vi "interface.vi"() -> ()   [LabVIEW 2016, in "Alarm interface.lvlib"]
uses:
  Alarm interface.lvlib
  WxMessage/wxpusher.lvlib
panel:
  in  "短信/语音设置":bool
  in  "微信设置":bool
  in  "报警定义":bool
  out "报警内容":string
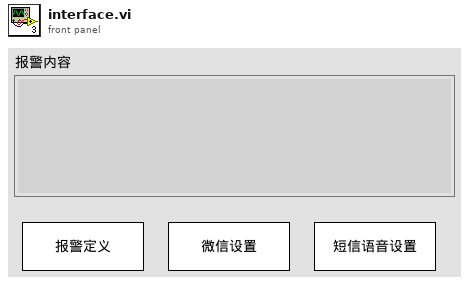
[diagram p1: front panel]
types:
  T1 = cluster{"报警模块":string, "告警码":string, "告警内容":string}
  T2 = enum32{"Invalid", "Standard", "Closed", "Hidden", "Minimized", "Maximized"}
  T3 = enum32{"Bad", "Idle", "Run top level", "Running"}
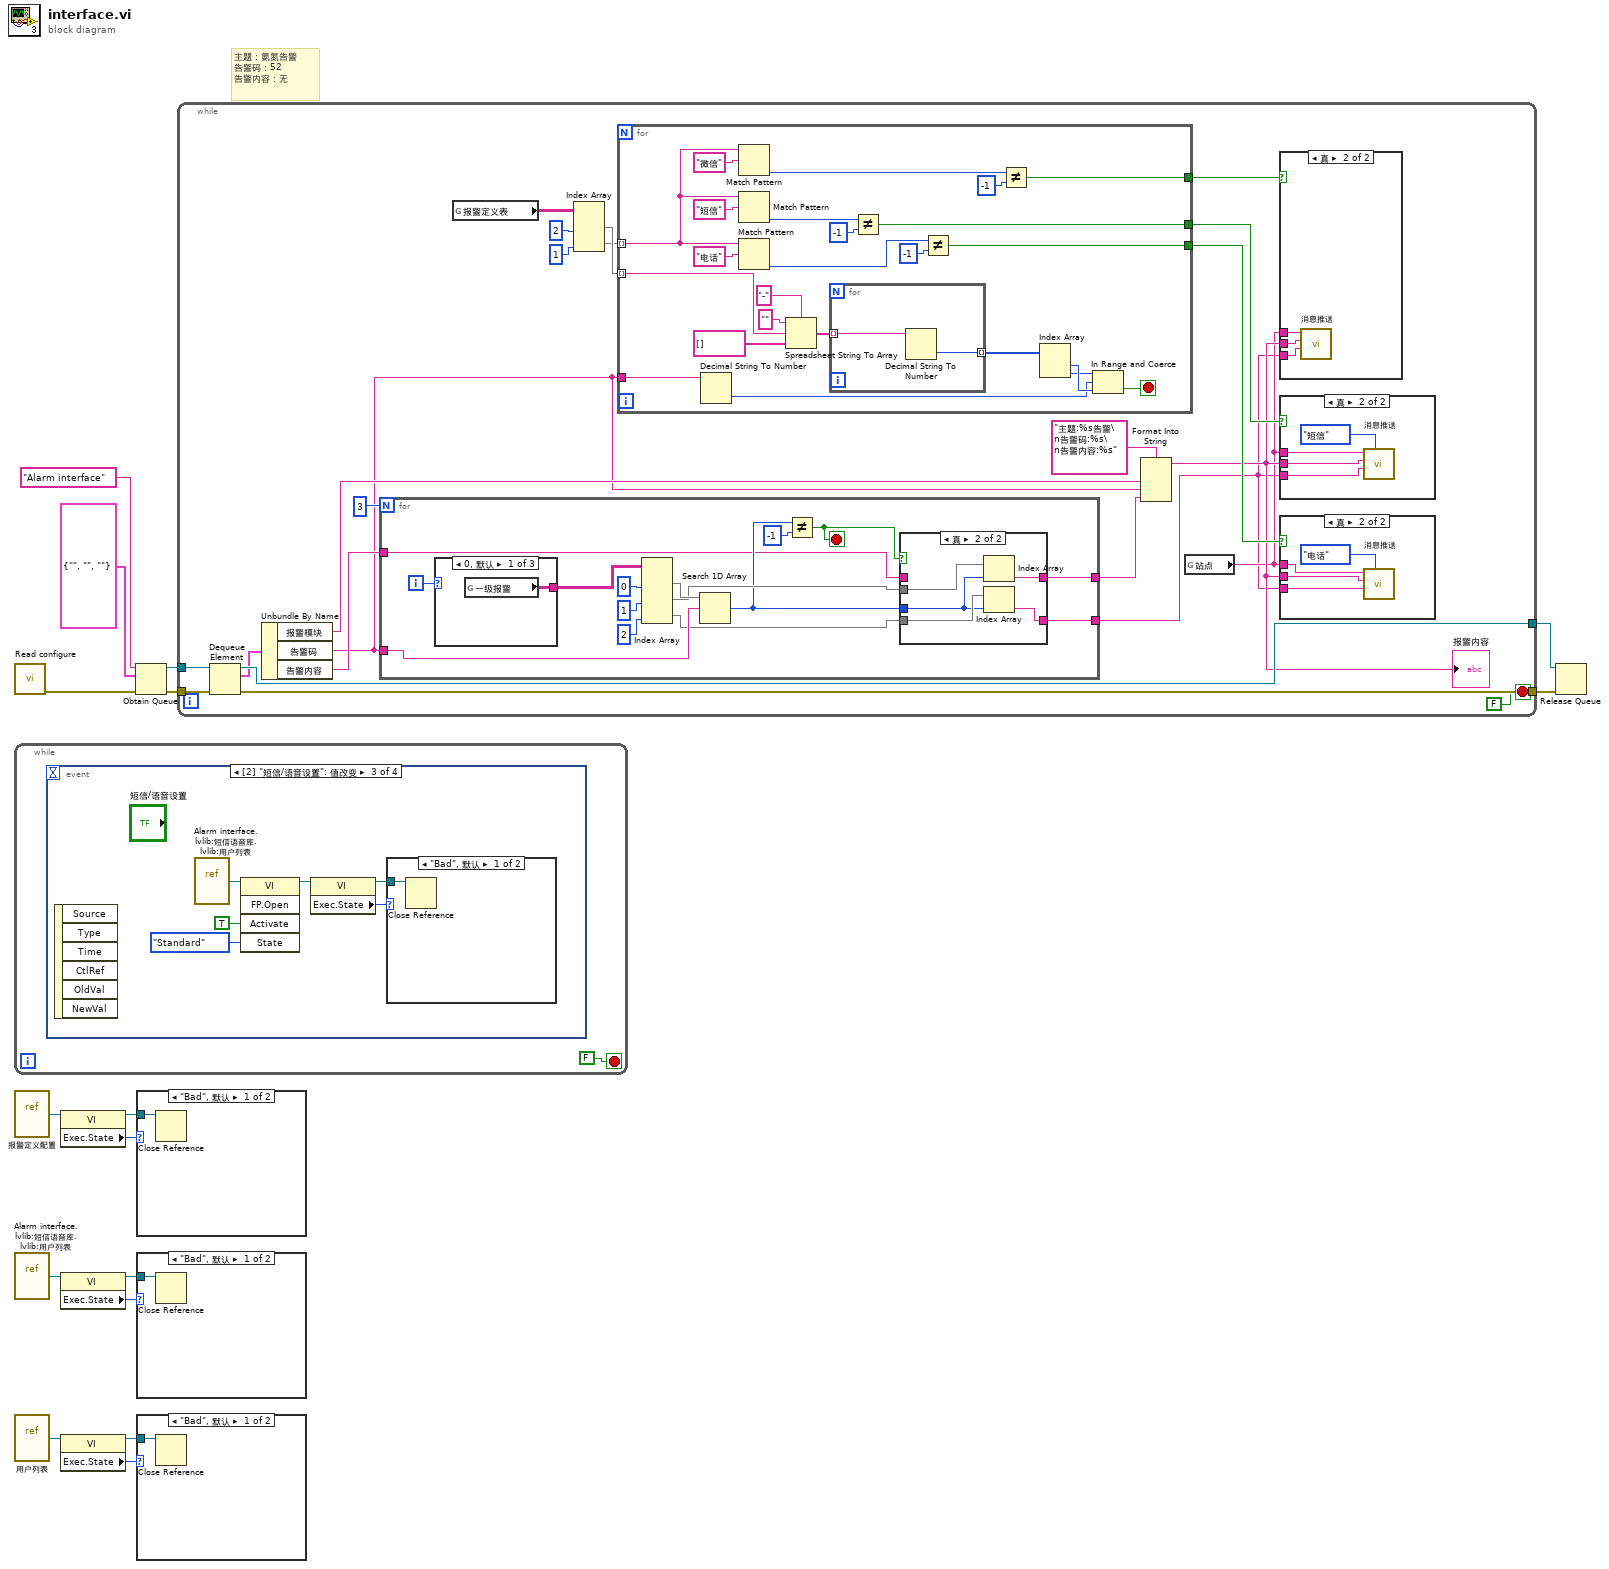
[diagram p0: block diagram]
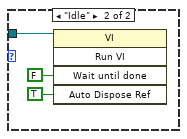
[diagram p2: hidden frame]
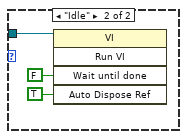
[diagram p3: hidden frame]
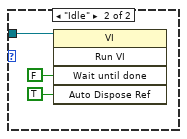
[diagram p4: hidden frame]
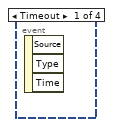
[diagram p5: hidden frame]
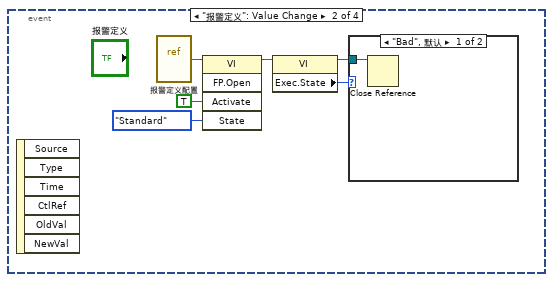
[diagram p6: hidden frame]
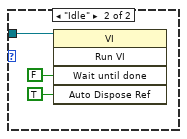
[diagram p7: hidden frame]
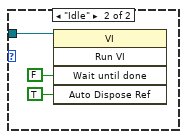
[diagram p8: hidden frame]
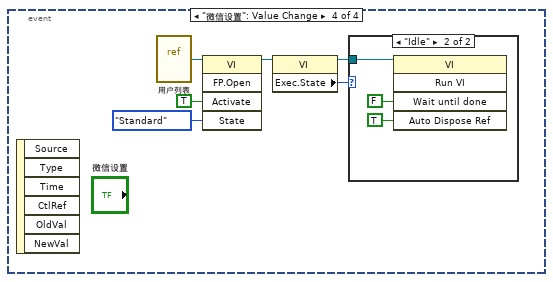
[diagram p9: hidden frame]
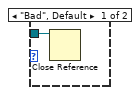
[diagram p10: hidden frame]
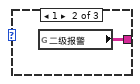
[diagram p14: hidden frame]
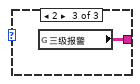
[diagram p15: hidden frame]
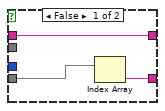
[diagram p16: hidden frame]
diagram:
  # "主题：氨氮告警\n告警码：52\n告警内容：无"
  n1 = call "Read configure.vi"() -> ("error out"=w10:errorcluster)  [unwired: 11 in]
  n2 = while {
    stop <- FALSE stop-if-true
    n3 = event shown="[2] \"短信/语音设置\": 值改变" {
      selector: _ -> [_ _ _ _]
      dyn-events: _ -> [_ _ _ _]
      timeout: _ -> [_ _ _ _]
      event Timeout {
        n4 = event-data() -> ()  [unwired: 1 in, 3 out]
      }
      event "报警定义": Value Change {
        n5 = event-data() -> ()  [unwired: 1 in, 6 out]
        n6 = vi-ref "报警定义配置.vi"() -> (w23:refnum<vi>)
        n7 = invoke class="VI" method="FP.Open"(reference=w23, "Activate"=TRUE ("激活？"), "State"=T2."Standard" ("状态")) -> (reference out=w20:refnum<vi>)  [unwired: 2 in, 4 out]
        n8 = property class="VI"(reference=w20) -> (reference out=w18:refnum<vi>, "Exec.State"=w19:T3)  [unwired: 1 in, 1 out]
        n9 = case shown="\"Bad\", 默认" w19 {
          tunnel: w18 -> [w24 w25]
          frame "Bad", Default {
            n10 = Close Reference(reference=w24) -> ()  [unwired: 1 in, 1 out]
          }
          frame "Idle" {
            n11 = invoke class="VI" method="Run VI"(reference=w25, "Wait until done"=FALSE ("结束前等待"), "Auto Dispose Ref"=TRUE ("自动销毁引用")) -> ()  [unwired: 2 in, 5 out]
          }
        }
      }
      event "短信/语音设置": Value Change {
        n12 = event-data() -> ()  [unwired: 1 in, 6 out]
        n13 = vi-ref "Alarm interface.lvlib:短信语音库.lvlib:用户列表.vi"() -> (w28:refnum<vi>)
        n14 = invoke class="VI" method="FP.Open"(reference=w28, "Activate"=TRUE ("激活？"), "State"=T2."Standard" ("状态")) -> (reference out=w31:refnum<vi>)  [unwired: 2 in, 4 out]
        n15 = property class="VI"(reference=w31) -> (reference out=w29:refnum<vi>, "Exec.State"=w30:T3)  [unwired: 1 in, 1 out]
        n16 = case shown="\"Bad\", 默认" w30 {
          tunnel: w29 -> [w34 w35]
          frame "Bad", Default {
            n17 = Close Reference(reference=w34) -> ()  [unwired: 1 in, 1 out]
          }
          frame "Idle" {
            n18 = invoke class="VI" method="Run VI"(reference=w35, "Wait until done"=FALSE ("结束前等待"), "Auto Dispose Ref"=TRUE ("自动销毁引用")) -> ()  [unwired: 2 in, 5 out]
          }
        }
      }
      event "微信设置": Value Change {
        n19 = event-data() -> ()  [unwired: 1 in, 6 out]
        n20 = vi-ref "用户列表.vi"() -> (w43:refnum<vi>)
        n21 = invoke class="VI" method="FP.Open"(reference=w43, "Activate"=TRUE ("激活？"), "State"=T2."Standard" ("状态")) -> (reference out=w40:refnum<vi>)  [unwired: 2 in, 4 out]
        n22 = property class="VI"(reference=w40) -> (reference out=w38:refnum<vi>, "Exec.State"=w39:T3)  [unwired: 1 in, 1 out]
        n23 = case shown="\"Idle\"" w39 {
          tunnel: w38 -> [w44 w45]
          frame "Bad", Default {
            n24 = Close Reference(reference=w44) -> ()  [unwired: 1 in, 1 out]
          }
          frame "Idle" {
            n25 = invoke class="VI" method="Run VI"(reference=w45, "Wait until done"=FALSE ("结束前等待"), "Auto Dispose Ref"=TRUE ("自动销毁引用")) -> ()  [unwired: 2 in, 5 out]
          }
        }
      }
    }
  }
  n26 = vi-ref "报警定义配置.vi"() -> (w7:refnum<vi>)
  n27 = vi-ref "Alarm interface.lvlib:短信语音库.lvlib:用户列表.vi"() -> (w4:refnum<vi>)
  n28 = vi-ref "用户列表.vi"() -> (w1:refnum<vi>)
  n29 = property class="VI"(reference=w7) -> (reference out=w8:refnum<vi>, "Exec.State"=w9:T3)  [unwired: 1 in, 1 out]
  n30 = property class="VI"(reference=w4) -> (reference out=w5:refnum<vi>, "Exec.State"=w6:T3)  [unwired: 1 in, 1 out]
  n31 = property class="VI"(reference=w1) -> (reference out=w2:refnum<vi>, "Exec.State"=w3:T3)  [unwired: 1 in, 1 out]
  n32 = Obtain Queue(name (unnamed)="Alarm interface" ("名称（未命名）"), element data type=T1 {"报警模块"="", "告警码"="", "告警内容"=""}, error in (no error)=w10) -> (queue out=w16:refnum<queue>, error out=w15:errorcluster)  [unwired: 2 in, 1 out]
  n33 = case shown="\"Bad\", 默认" w9 {
    tunnel: w8 -> [w48 w49]
    frame "Bad", Default {
      n34 = Close Reference(reference=w48) -> ()  [unwired: 1 in, 1 out]
    }
    frame "Idle" {
      n35 = invoke class="VI" method="Run VI"(reference=w49, "Wait until done"=FALSE ("结束前等待"), "Auto Dispose Ref"=TRUE ("自动销毁引用")) -> ()  [unwired: 2 in, 5 out]
    }
  }
  n36 = case shown="\"Bad\", 默认" w6 {
    tunnel: w5 -> [w52 w53]
    frame "Bad", Default {
      n37 = Close Reference(reference=w52) -> ()  [unwired: 1 in, 1 out]
    }
    frame "Idle" {
      n38 = invoke class="VI" method="Run VI"(reference=w53, "Wait until done"=FALSE ("结束前等待"), "Auto Dispose Ref"=TRUE ("自动销毁引用")) -> ()  [unwired: 2 in, 5 out]
    }
  }
  n39 = case shown="\"Bad\", 默认" w3 {
    tunnel: w2 -> [w56 w57]
    frame "Bad", Default {
      n40 = Close Reference(reference=w56) -> ()  [unwired: 1 in, 1 out]
    }
    frame "Idle" {
      n41 = invoke class="VI" method="Run VI"(reference=w57, "Wait until done"=FALSE ("结束前等待"), "Auto Dispose Ref"=TRUE ("自动销毁引用")) -> ()  [unwired: 2 in, 5 out]
    }
  }
  n42 = while {
    tunnel: w16 -> [w82]
    tunnel: w15 -> [w81]
    tunnel: [w80] -> w14
    tunnel: [w79] -> w13
    stop <- FALSE stop-if-true
    n43 = Dequeue Element(queue=w82, error in (no error)=w81) -> (queue out=w80:refnum<queue>, element=w77:T1, error out=w79:errorcluster)  [unwired: 1 in, 1 out]
    n44 = Unbundle By Name(w77) -> ("报警模块"=w75:string, "告警码"=w66:string, "告警内容"=w74:string)
    n45 = for {
      N: 3 -> [_]
      tunnel: w66 -> [w127]
      tunnel: w74 -> [w126]
      tunnel: [w123] -> w72
      tunnel: [w120] -> w60
      i -> [w125]
      stop <- w124 stop-if-true
      n46 = case shown="0, 默认" w125 {
        tunnel: [w135 w136 w137] -> w132
        frame 0, Default {
          n47 = global read "断电保存全局.vi" "一级报警"() -> (w135:string[][])
        }
        frame 1 {
          n48 = global read "断电保存全局.vi" "二级报警"() -> (w136:string[][])
        }
        frame 2 {
          n49 = global read "断电保存全局.vi" "三级报警"() -> (w137:string[][])
        }
      }
      n50 = Index Array(array=w132, index (col) #1=0 ("禁用的索引 (列)"), index (col) #2=1 ("索引 (列)"), index (col) #3=2 ("索引 (列)")) -> (element #1=w134:string[], element #2=w129:string[], element #3=w121:string[])  [unwired: 3 in]
      n51 = Search 1D Array(1D array=w134, element=w127) -> (index of element=w128:i32)  [unwired: 1 in]
      n52 = Not Equal?(x=w128, y=-1) -> (x != y?=w124:bool)
      n53 = case shown="真" w124 {
        tunnel: w129 -> [_ w145]
        tunnel: w128 -> [_ w142]
        tunnel: [w140 w144] -> w123
        tunnel: w126 -> [w140 _]
        tunnel: w121 -> [w139 w143]
        tunnel: [w138 w141] -> w120
        frame False {
          n54 = Index Array(array=w139) -> (element=w138:string)  [unwired: 1 in]
        }
        frame True {
          n55 = Index Array(array=w145, index=w142) -> (element=w144:string)
          n56 = Index Array(array=w143, index=w142) -> (element=w141:string)
        }
      }
    }
    n57 = global read "断电保存全局.vi" "报警定义表"() -> (w71:string[][])
    n58 = Index Array(array=w71, index (col) #1=2 ("禁用的索引 (列)"), index (col) #2=1 ("索引 (列)")) -> (element #1=w69:string[], element #2=w67:string[])  [unwired: 2 in]
    n59 = for {
      tunnel: w69 -> [w112] mode=indexing
      tunnel: w67 -> [w99] mode=indexing
      tunnel: [w98] -> w65
      tunnel: [w97] -> w63
      tunnel: [w96] -> w64
      tunnel: w66 -> [w95]
      stop <- w109 stop-if-true
      n60 = Decimal String To Number(string=w95) -> (number=w94:i32)  [unwired: 2 in, 1 out]
      n61 = Match Pattern(string=w99, regular expression="微信" ("正则表达式")) -> (offset past match=w101:i32)  [unwired: 1 in, 3 out]
      n62 = Match Pattern(string=w99, regular expression="短信" ("正则表达式")) -> (offset past match=w107:i32)  [unwired: 1 in, 3 out]
      n63 = Match Pattern(string=w99, regular expression="电话" ("正则表达式")) -> (offset past match=w104:i32)  [unwired: 1 in, 3 out]
      n64 = Spreadsheet String To Array(delimiter (Tab)="-" ("分隔符(Tab)"), format string="" ("格式字符串"), spreadsheet string=w112, array type (2D Dbl)=string[] []) -> (array=w114:string[])
      n65 = for {
        tunnel: w114 -> [w119] mode=indexing
        tunnel: [w118] -> w113 mode=indexing
        n66 = Decimal String To Number(string=w119) -> (number=w118:i32)  [unwired: 2 in, 1 out]
      }
      n67 = Not Equal?(x=w107, y=-1) -> (x != y?=w98:bool)
      n68 = Not Equal?(x=w104, y=-1) -> (x != y?=w97:bool)
      n69 = Not Equal?(x=w101, y=-1) -> (x != y?=w96:bool)
      n70 = Index Array(array=w113) -> (element #1=w111:i32, element #2=w110:i32)  [unwired: 2 in]
      n71 = In Range and Coerce(upper limit=w110, x=w94, lower limit=w111) -> (In Range?=w109:bool)  [unwired: 1 out]
    }
    n72 = Format Into String(format string="主题:%s告警\n告警码:%s\n告警内容:%s" ("格式字符串"), w75, w66, w72) -> (resulting string=w62:string)  [unwired: 2 in, 1 out]
    "报警内容" <- w62
    n73 = global read "短信服务全局变量.vi" "站点"() -> (w61:string)
    n74 = case shown="真" w64 {
      tunnel: w62 -> [_ w89]
      tunnel: w61 -> [_ w88]
      tunnel: w60 -> [_ w87]
      frame False {
      }
      frame True {
        n75 = call "消息推送.vi"("分析"=w87, "内容"=w89, "站点"=w88) -> ()  [unwired: 8 in, 1 out]
      }
    }
    n76 = case shown="真" w65 {
      tunnel: w62 -> [_ w93]
      tunnel: w61 -> [_ w92]
      tunnel: w60 -> [_ w90]
      frame False {
      }
      frame True {
        n77 = call "消息推送.vi"("枚举"=enum16{"短信", "电话"}."短信", "分析"=w90, "内容"=w93, "站点"=w92) -> ()  [unwired: 7 in, 1 out]
      }
    }
    n78 = case shown="真" w63 {
      tunnel: w62 -> [_ w86]
      tunnel: w61 -> [_ w85]
      tunnel: w60 -> [_ w83]
      frame False {
      }
      frame True {
        n79 = call "消息推送.vi"("枚举"=enum16{"短信", "电话"}."电话", "分析"=w83, "内容"=w86, "站点"=w85) -> ()  [unwired: 7 in, 1 out]
      }
    }
  }
  n80 = Release Queue(queue=w14, error in (no error)=w13) -> ()  [unwired: 1 in, 3 out]
